vi "CalibrationState.vi"() -> ()   [LabVIEW 2012]
panel:
  in  "CalibrationState":T1
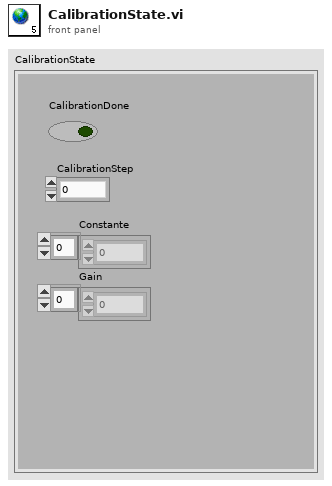
[diagram p1: front panel]
types:
  T1 = cluster{"CalibrationDone":bool, "CalibrationStep":u32, "Constante":dbl[], "Gain":dbl[]}
diagram:
